vi "draw.vi"(0 "reference in":refnum<class "DQMHModuleNode.lvclass">, 1 "graphics":refnum<class "Graphics.lvclass">, 5 "error in (no error)":errorcluster) -> (14 "reference out":refnum<class "DQMHModuleNode.lvclass">, 19 "error out":errorcluster)   [LabVIEW 2016, in "DQMHModuleNode.lvclass"]
doc: "public void draw(Graphics2D g2, Point2D p, Point2D q)"
uses:
  <resource>/Framework/Providers/Open_GDS/UML/DQMHModuleNode_class/DQMHModuleNode.lvclass
  C:/Program Files (x86)/National Instruments/LabVIEW 2016/resource/Framework/Providers/Open_GDS/UML/RectangularNode_class/RectangularNode.lvclass
  <resource>/Framework/Providers/Open_GDS/UML/Graphics_class/Graphics.lvclass
  <resource>/Framework/Providers/Open_GDS/UML/General/Rectangle/Rectangle Rectangle2D.ctl
  <resource>/Framework/Providers/Open_GDS/UML/MultiLineString_class/MultiLineString.lvclass
  <resource>/Framework/Providers/Open_GDS/UML/RectangularNode_class/RectangularNode.lvclass
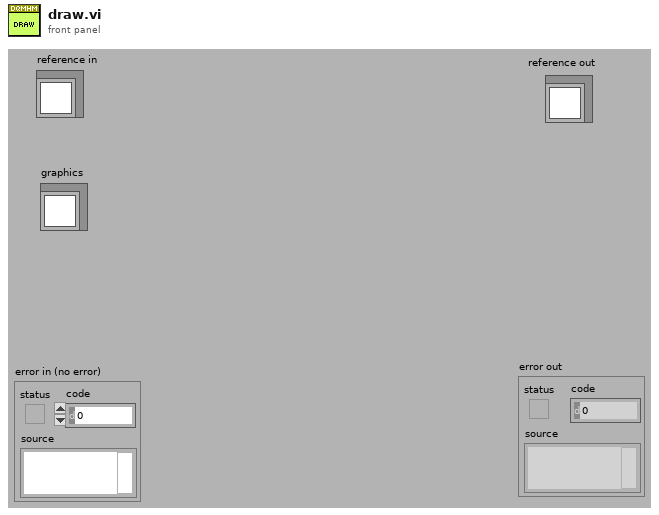
[diagram p1: front panel]
types:
  T1 = typedef "Rectangle Rectangle2D.ctl" = cluster{"x":dbl, "y":dbl, "width":dbl, "height":dbl}
  T2 = typedef "DQMHModuleNode.lvclass/ObjectAttributes.ctl" = cluster{"DescriptionHeight":dbl, "InternalDataHeight":dbl, "EventsHeight":dbl, "Name":refnum<class "MultiLineString.lvclass">, "Description":refnum<class "MultiLineString.lvclass">, "InternalData":refnum<class "MultiLineString.lvclass">, "Events":refnum<class "MultiLineString.lvclass">, "showDescription":bool, "showInternalData":bool, "showEvents":bool, "DEFAULT_ROUNDING":i32, "DEFAULT_WIDTH":i32, "DEFAULT_HEIGHT":i32, "ClassPath":path, "Template":string, "Icon":u8[][]}
  T3 = typedef "RectangularNode.lvclass/ObjectAttributes.ctl" = cluster{"bounds":T1}
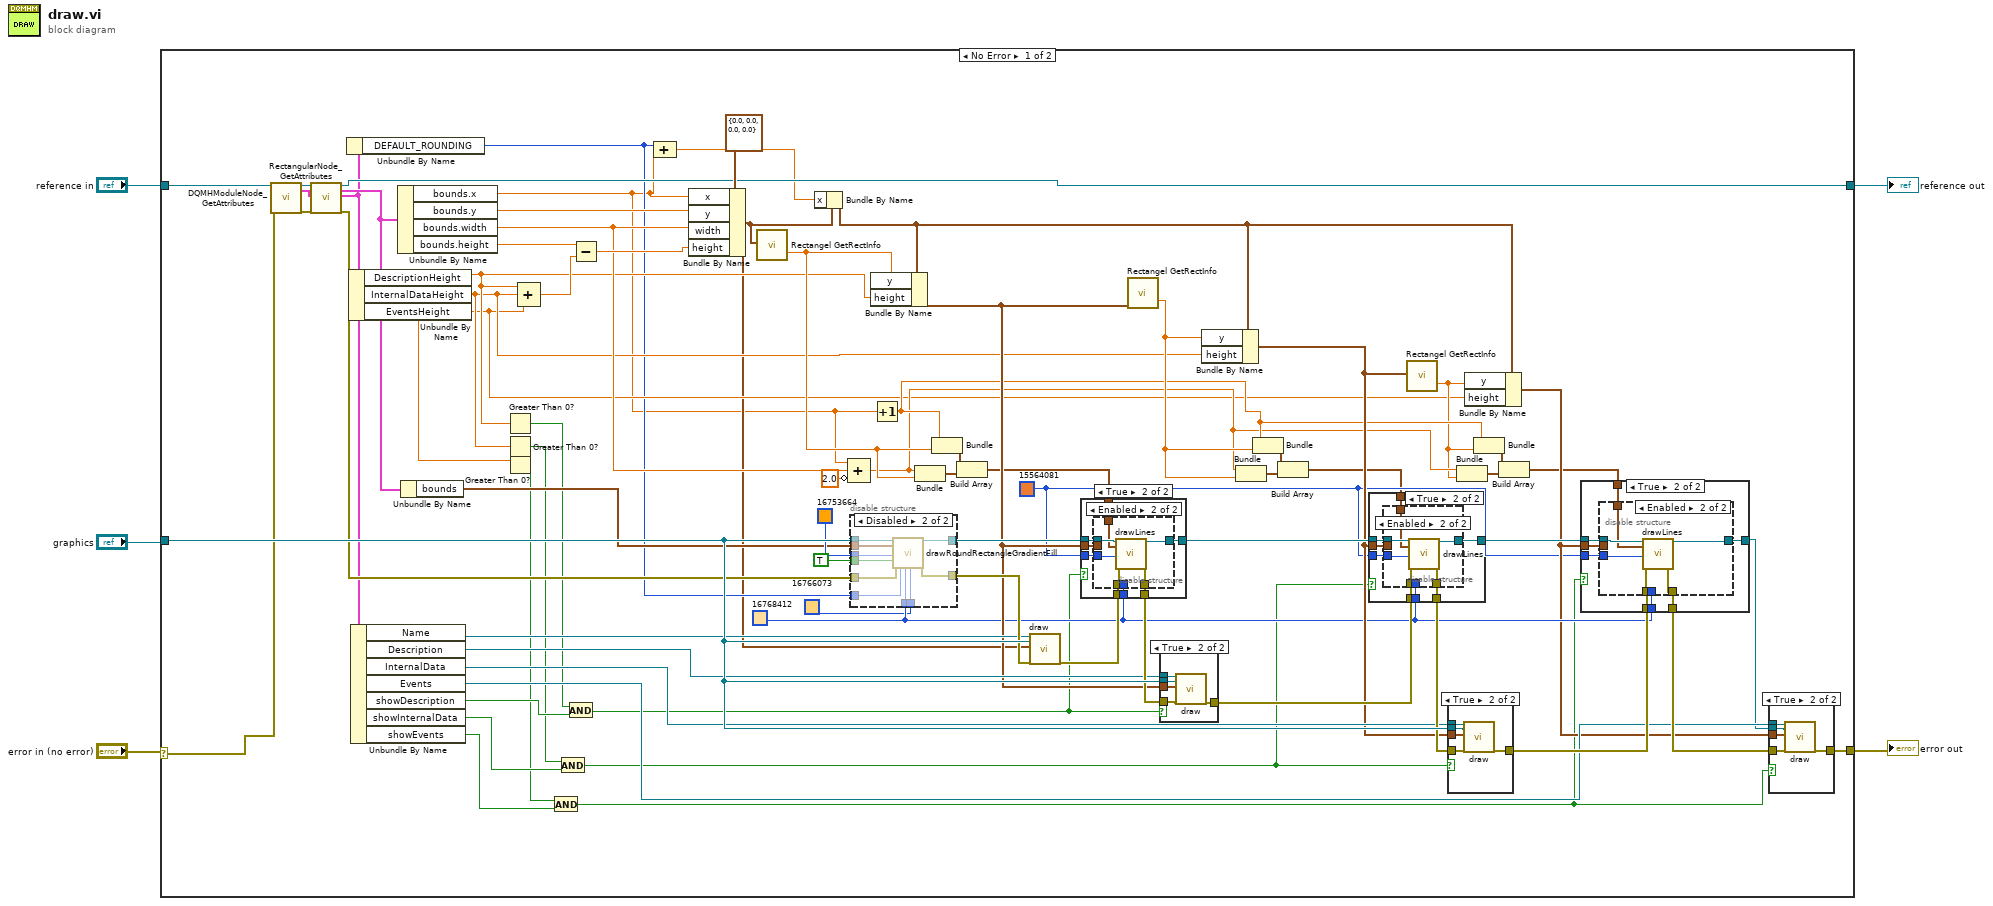
[diagram p0: block diagram]
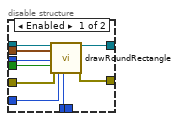
[diagram p2: hidden frame]
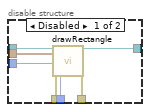
[diagram p5: hidden frame]
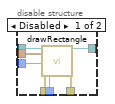
[diagram p7: hidden frame]
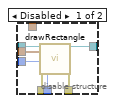
[diagram p9: hidden frame]
diagram:
  n1 = case shown="No Error" "error in (no error)" {
    selector: "error in (no error)" -> [w75 w184]
    tunnel: "reference in" -> [w77 w185]
    tunnel: [w52 w184] -> w4
    tunnel: [w56 w185] -> w3
    tunnel: "graphics" -> [w76 _]
    frame No Error {
      w34 = u32 15564081
      w43 = u32 16768412
      n2 = call <resource>:"DQMHModuleNode_GetAttributes.vi"("reference in"=w77, "error in (no error)"=w75) -> ("reference out"=w58:refnum<class "DQMHModuleNode.lvclass">, "Data"=w12:T2, "error out"=w57:errorcluster)  [unwired: 1 in, 14 out]
      n3 = call <resource>:"RectangularNode_GetAttributes.vi"("reference in"=w58, "error in (no error)"=w57) -> ("reference out"=w56:refnum<class "DQMHModuleNode.lvclass">, "Data"=w23:T3, "error out"=w55:errorcluster)  [unwired: 14 in, 1 out]
      n4 = Unbundle By Name(w12) -> ("DEFAULT_ROUNDING"=w11:i32)
      n5 = Unbundle By Name(w12) -> ("DescriptionHeight"=w18:dbl, "InternalDataHeight"=w14:dbl, "EventsHeight"=w13:dbl)
      n6 = Unbundle By Name(w12) -> ("Name"=w60:refnum<class "MultiLineString.lvclass">, "Description"=w61:refnum<class "MultiLineString.lvclass">, "InternalData"=w62:refnum<class "MultiLineString.lvclass">, "Events"=w50:refnum<class "MultiLineString.lvclass">, "showDescription"=w47:bool, "showInternalData"=w46:bool, "showEvents"=w45:bool)
      n7 = Unbundle By Name(w23) -> ("bounds.x"=w7:dbl, "bounds.y"=w71:dbl, "bounds.width"=w37:dbl, "bounds.height"=w73:dbl)
      n8 = Unbundle By Name(w23) -> ("bounds"=w22:T1)
      n9 = Greater Than 0?(x=w18) -> (x > 0?=w17:bool)
      n10 = Greater Than 0?(x=w14) -> (x > 0?=w16:bool)
      n11 = Greater Than 0?(x=w13) -> (x > 0?=w15:bool)
      n12 = Compound Arithmetic op=ADD(w18, w14, w13) -> (w70:dbl)
      n13 = And(x=w15, y=w45) -> (x .and. y?=w19:bool)
      n14 = And(x=w16, y=w46) -> (x .and. y?=w20:bool)
      n15 = And(x=w17, y=w47) -> (x .and. y?=w21:bool)
      n16 = Subtract(x=w73, y=w70) -> (x-y=w72:dbl)
      n17 = Compound Arithmetic op=ADD(w11, w7) -> (w8:dbl)
      n18 = Bundle By Name(cluster=T1 {"x"=0.0, "y"=0.0, "width"=0.0, "height"=0.0} ("points"), "x"=w7, "y"=w71, "width"=w37, "height"=w72) -> (w10:T1)
      n19 = call <resource>:"Rectangel GetRectInfo.vi"("bounds"=w10) -> ("maxY"=w35:dbl)  [unwired: 1 in, 17 out]
      n20 = Bundle By Name(cluster=w10, "x"=w8) -> (w9:T1)
      n21 = Compound Arithmetic op=ADD(w7, w37, invert 2.0 ("value")) -> (w26:dbl)
      n22 = disable-structure shown="Disabled" {
        disable-tunnel: w76 -> [w86 w96]
        disable-tunnel: [w85 w95] -> w69
        disable-tunnel: [w84 w94] -> w67
        disable-tunnel: w55 -> [w83 w93]
        disable-tunnel: u32 16753664 -> [w82 w92]
        disable-tunnel: w43 -> [w81 w91]
        disable-tunnel: TRUE ("fill?(F)") -> [w80 w90]
        disable-tunnel: w22 -> [w79 w89]
        disable-tunnel: w11 -> [w78 w88]
        disable-tunnel: u32 16766073 ("Color Box") -> [_ w87]
        frame Enabled {
          n23 = call-dynamic "drawRoundRectangle.vi"("reference"=w86, "rectangle"=w79, "color(if not used=default color)"=w82, "fill?(F)"=w80, "error in (no error)"=w83, "RoundRadius"=w78, "FillClor(if not used=BorderColorIsUsed,AutoFill)"=w81) -> ("reference out"=w85:refnum<class "Graphics.lvclass">, "error out"=w84:errorcluster)  [unwired: 11 in]
        }
        frame Disabled {
          n24 = call-dynamic "drawRoundRectangleGradientFill.vi"("reference"=w96, "rectangle"=w89, "color(if not used=default color)"=w92, "fill?(F)"=w90, "error in (no error)"=w93, "RoundRadius"=w88, "TopFillColor"=w91, "BottomFillColor"=w87) -> ("reference out"=w95:refnum<class "Graphics.lvclass">, "error out"=w94:errorcluster)  [unwired: 10 in]
        }
      }
      n25 = Bundle By Name(cluster=w9, "y"=w35, "height"=w18) -> (w59:T1)
      n26 = Increment(x=w7) -> (x+1=w27:dbl)
      n27 = Bundle(w26, "maxY"=w35) -> (w38:cluster{dbl, "maxY":dbl})  [unwired: 1 in]
      n28 = Bundle(w27, "maxY"=w35) -> (w40:cluster{dbl, "maxY":dbl})  [unwired: 1 in]
      n29 = Build Array(w40, w38) -> (w39:cluster{dbl, "maxY":dbl}[])
      n30 = call-dynamic "draw.vi"("reference"=w60, "graphics"=w76, "bounds"=w10, "error in (no error)"=w67) -> ("error out"=w66:errorcluster)  [unwired: 14 in, 1 out]
      n31 = case shown="True" w21 {
        tunnel: w69 -> [w150 w158]
        tunnel: [w150 w157] -> w68
        tunnel: w66 -> [w149 w156]
        tunnel: [w149 w155] -> w65
        tunnel: w43 -> [_ w154]
        tunnel: w59 -> [_ w153]
        tunnel: w34 -> [_ w152]
        tunnel: w39 -> [_ w151]
        frame False {
        }
        frame True {
          n32 = disable-structure shown="Enabled" {
            disable-tunnel: w158 -> [w165 w169]
            disable-tunnel: [w164 w168] -> w157
            disable-tunnel: w156 -> [w163 w171]
            disable-tunnel: [w162 w170] -> w155
            disable-tunnel: w154 -> [w161 _]
            disable-tunnel: w153 -> [w160 _]
            disable-tunnel: w152 -> [w159 w166]
            disable-tunnel: w151 -> [_ w167]
            frame Disabled {
              n33 = call <resource>:"drawRectangle.vi"("reference"=w165, "rectangle"=w160, "color(if not used=default color)"=w159, "error in (no error)"=w163, "FillClor(if not used=BorderColorIsUsed,AutoFill)"=w161) -> ("reference out"=w164:refnum<class "Graphics.lvclass">, "error out"=w162:errorcluster)  [unwired: 2 in, 11 out]
            }
            frame Enabled {
              n34 = call <resource>:"drawLines.vi"("reference"=w169, "points"=w167, "color(if not used=default color)"=w166, "error in (no error)"=w171) -> ("reference out"=w168:refnum<class "Graphics.lvclass">, "error out"=w170:errorcluster)  [unwired: 14 in]
            }
          }
        }
      }
      n35 = call <resource>:"Rectangel GetRectInfo.vi"("bounds"=w59) -> ("maxY"=w31:dbl)  [unwired: 1 in, 17 out]
      n36 = case shown="True" w21 {
        tunnel: w65 -> [w178 w183]
        tunnel: [w178 w182] -> w64
        tunnel: w61 -> [_ w181]
        tunnel: w76 -> [_ w180]
        tunnel: w59 -> [_ w179]
        frame False {
        }
        frame True {
          n37 = call-dynamic "draw.vi"("reference"=w181, "graphics"=w180, "bounds"=w179, "error in (no error)"=w183) -> ("error out"=w182:errorcluster)  [unwired: 14 in, 1 out]
        }
      }
      n38 = Bundle By Name(cluster=w9, "y"=w31, "height"=w14) -> (w48:T1)
      n39 = Bundle(w26, "maxY"=w31) -> (w33:cluster{dbl, "maxY":dbl})  [unwired: 1 in]
      n40 = Bundle(w27, "maxY"=w31) -> (w32:cluster{dbl, "maxY":dbl})  [unwired: 1 in]
      n41 = Build Array(w32, w33) -> (w30:cluster{dbl, "maxY":dbl}[])
      n42 = case shown="True" w20 {
        tunnel: w68 -> [w126 w135]
        tunnel: w64 -> [w127 w134]
        tunnel: [w127 w133] -> w63
        tunnel: w43 -> [_ w132]
        tunnel: w48 -> [_ w131]
        tunnel: [w126 w130] -> w54
        tunnel: w34 -> [_ w129]
        tunnel: w30 -> [_ w128]
        frame False {
        }
        frame True {
          n43 = disable-structure shown="Enabled" {
            disable-tunnel: w135 -> [w142 w148]
            disable-tunnel: w134 -> [w141 w146]
            disable-tunnel: [w140 w145] -> w133
            disable-tunnel: w132 -> [w139 _]
            disable-tunnel: w131 -> [w138 _]
            disable-tunnel: [w137 w147] -> w130
            disable-tunnel: w129 -> [w136 w144]
            disable-tunnel: w128 -> [_ w143]
            frame Disabled {
              n44 = call <resource>:"drawRectangle.vi"("reference"=w142, "rectangle"=w138, "color(if not used=default color)"=w136, "error in (no error)"=w141, "FillClor(if not used=BorderColorIsUsed,AutoFill)"=w139) -> ("reference out"=w137:refnum<class "Graphics.lvclass">, "error out"=w140:errorcluster)  [unwired: 2 in, 11 out]
            }
            frame Enabled {
              n45 = call <resource>:"drawLines.vi"("reference"=w148, "points"=w143, "color(if not used=default color)"=w144, "error in (no error)"=w146) -> ("reference out"=w147:refnum<class "Graphics.lvclass">, "error out"=w145:errorcluster)  [unwired: 14 in]
            }
          }
        }
      }
      n46 = call <resource>:"Rectangel GetRectInfo.vi"("bounds"=w48) -> ("maxY"=w25:dbl)  [unwired: 1 in, 17 out]
      n47 = case shown="True" w20 {
        tunnel: w63 -> [w172 w177]
        tunnel: [w172 w176] -> w53
        tunnel: w62 -> [_ w175]
        tunnel: w76 -> [_ w174]
        tunnel: w48 -> [_ w173]
        frame False {
        }
        frame True {
          n48 = call-dynamic "draw.vi"("reference"=w175, "graphics"=w174, "bounds"=w173, "error in (no error)"=w177) -> ("error out"=w176:errorcluster)  [unwired: 14 in, 1 out]
        }
      }
      n49 = Bundle(w26, "maxY"=w25) -> (w28:cluster{dbl, "maxY":dbl})  [unwired: 1 in]
      n50 = Bundle By Name(cluster=w9, "y"=w25, "height"=w13) -> (w41:T1)
      n51 = Bundle(w27, "maxY"=w25) -> (w29:cluster{dbl, "maxY":dbl})  [unwired: 1 in]
      n52 = Build Array(w29, w28) -> (w24:cluster{dbl, "maxY":dbl}[])
      n53 = case shown="True" w19 {
        tunnel: w54 -> [w103 w112]
        tunnel: w53 -> [w104 w111]
        tunnel: [w104 w110] -> w51
        tunnel: w41 -> [_ w109]
        tunnel: [w103 w108] -> w49
        tunnel: w34 -> [_ w107]
        tunnel: w43 -> [_ w106]
        tunnel: w24 -> [_ w105]
        frame False {
        }
        frame True {
          n54 = disable-structure shown="Enabled" {
            disable-tunnel: w112 -> [w119 w125]
            disable-tunnel: w111 -> [w118 w123]
            disable-tunnel: [w117 w122] -> w110
            disable-tunnel: w109 -> [w116 _]
            disable-tunnel: [w115 w124] -> w108
            disable-tunnel: w107 -> [w114 w121]
            disable-tunnel: w106 -> [w113 _]
            disable-tunnel: w105 -> [_ w120]
            frame Disabled {
              n55 = call <resource>:"drawRectangle.vi"("reference"=w119, "rectangle"=w116, "color(if not used=default color)"=w114, "error in (no error)"=w118, "FillClor(if not used=BorderColorIsUsed,AutoFill)"=w113) -> ("reference out"=w115:refnum<class "Graphics.lvclass">, "error out"=w117:errorcluster)  [unwired: 2 in, 11 out]
            }
            frame Enabled {
              n56 = call <resource>:"drawLines.vi"("reference"=w125, "points"=w120, "color(if not used=default color)"=w121, "error in (no error)"=w123) -> ("reference out"=w124:refnum<class "Graphics.lvclass">, "error out"=w122:errorcluster)  [unwired: 14 in]
            }
          }
        }
      }
      n57 = case shown="True" w19 {
        tunnel: w51 -> [w97 w102]
        tunnel: [w97 w101] -> w52
        tunnel: w50 -> [_ w100]
        tunnel: w49 -> [_ w99]
        tunnel: w41 -> [_ w98]
        frame False {
        }
        frame True {
          n58 = call-dynamic "draw.vi"("reference"=w100, "graphics"=w99, "bounds"=w98, "error in (no error)"=w102) -> ("error out"=w101:errorcluster)  [unwired: 14 in, 1 out]
        }
      }
    }
    frame Error {
    }
  }
  "reference out" <- w3
  "error out" <- w4
